vi "EncodeData.vi"(8 "Error In":errorcluster, 11 "Data In":u8[](array[numeric])) -> (0 "Error Out":errorcluster, 3 "Encoded Data Out":u8[](array[numeric]))   [LabVIEW 2010]
uses:
  RScode.dll
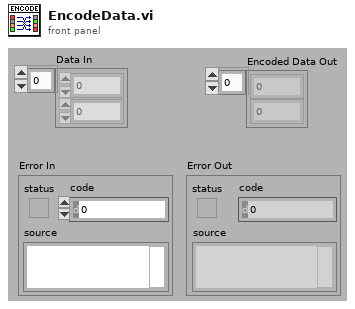
[diagram p1: front panel]
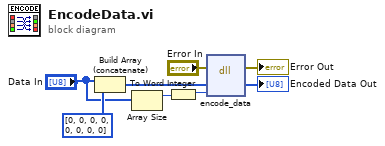
[diagram p0: block diagram]
diagram:
  n1 = Build Array (concatenate)("Data In", u8[] [0, 0, 0, 0, 0, 0, 0, 0] ("unsigned byte array")) -> (w7:u8[])
  n2 = Array Size(array="Data In") -> (size(s)=w5:i32)
  n3 = To Word Integer(number=w5) -> (16bit integer=w6:i16)
  n4 = dll-call lib="Z:/Ted On My Mac/GitHub/Configurator/Source/Utilities/RScode/RScode.dll" fn="encode_data"(error in="Error In", "msg"=w7, "nbytes"=w6) -> (error out=→"Error Out":errorcluster, "msg"=→"Encoded Data Out":u8[])  [unwired: 4 in, 1 out]
